vi "Single.vi"(8 "error in":errorcluster, 11 "com in":refnum<visa-resource-name>) -> (0 "error out":errorcluster, 2 "Data":i64[](array[numeric]), 3 "com out":refnum<visa-resource-name>)   [LabVIEW 2020]
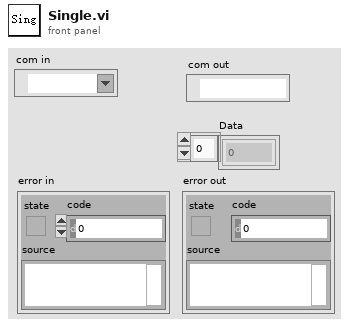
[diagram p1: front panel]
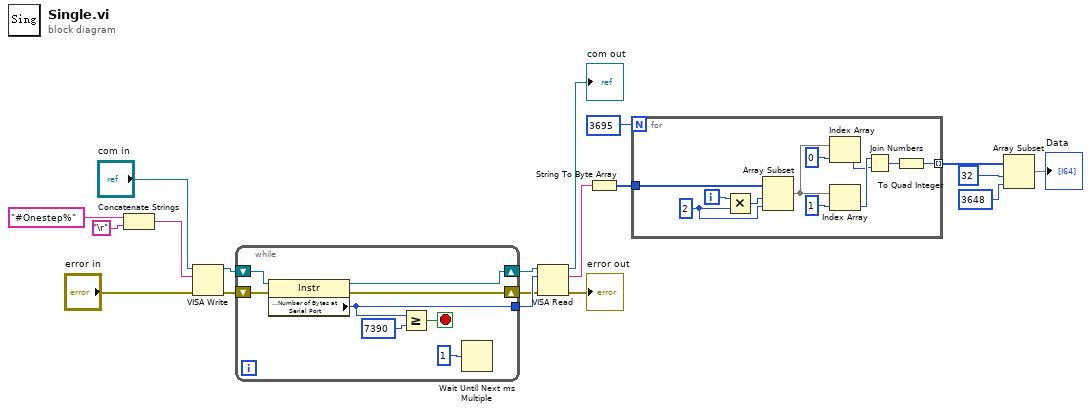
[diagram p0: block diagram]
diagram:
  n1 = Concatenate Strings("#Onestep%" ("字符串"), "\r") -> (w19:string)
  n2 = VISA Write(VISA resource name="com in", write buffer=w19, error in (no error)="error in") -> (VISA resource name out=w2:refnum<visa-resource-name>, error out=w3:errorcluster)  [unwired: 1 out]
  n3 = while {
    tunnel: [w23] -> w13
    shift-right: [w26] -> w12
    shift-left: w3 -> [w25]
    shift-right: [w27] -> w14
    shift-left: w2 -> [w24]
    stop <- w22 stop-if-true
    n4 = property class="Instr"(reference=w24, error in=w25) -> (reference out=w27:refnum<visa-resource-name>, error out=w26:errorcluster, "Serial Settings:Number of Bytes at Serial Port"=w23:u32)
    n5 = Greater Or Equal?(x=w23, y=u32 7390) -> (x >= y?=w22:bool)
    n6 = Wait Until Next ms Multiple(millisecond multiple=u32 1 ("毫秒倍数")) -> ()  [unwired: 1 out]
  }
  n7 = VISA Read(VISA resource name=w14, byte count=w13, error in (no error)=w12) -> (VISA resource name out=→"com out":refnum<visa-resource-name>, read buffer=w11:string, error out=→"error out":errorcluster)  [unwired: 1 out]
  n8 = String To Byte Array(string=w11) -> (unsigned byte array=w10:u8[])
  n9 = for {
    N: 3695 -> [_]
    tunnel: w10 -> [w38]
    tunnel: [w30] -> w8 mode=indexing
    i -> [w36]
    w35 = 2 ("长度")
    n10 = Multiply(x=w36, y=w35) -> (x*y=w37:i32)
    n11 = Array Subset(array=w38, index=w37, length=w35) -> (w34:u8[])
    n12 = Index Array(array=w34, index=0 ("索引")) -> (element=w28:u8)
    n13 = Index Array(array=w34, index=1 ("索引")) -> (element=w29:u8)
    n14 = Join Numbers(hi=w29, lo=w28) -> ((hi.lo)=w31:u16)
    n15 = To Quad Integer(1:w31) -> (0:w30:i64)
  }
  n16 = Array Subset(array=w8, index=32 ("索引"), length=3648 ("长度")) -> (→"Data":i64[])
